vi "Add New Waypoint.vi"(8 "Error In":errorcluster, 9 "Altitude (m)":sgl, 10 "Lon":sgl, 11 "Lat":sgl) -> (0 "Error Out":errorcluster)   [LabVIEW 2014]
uses:
  Aircraft Information/Sub VI/Selected Aircraft/SubVI/Get Selected Aircraft.vi
  Aircraft Information/Sub VI/Get Aircraft Waypoints.vi
  FGV/Methods/Get Waypoint type.vi
  Aircraft Information/Sub VI/Set Aircraft Waypoints.vi
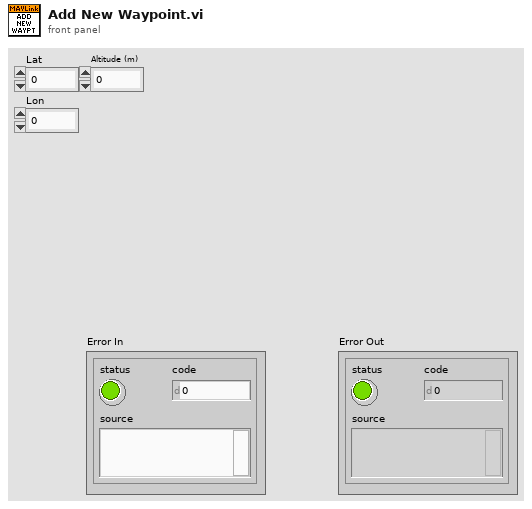
[diagram p1: front panel]
types:
  T1 = typedef "MAVLINK Mav Frame.ctl" = enum8{"GLOBAL", "LOCAL NED", "MISSION", "GLOBAL RELATIVE ALT", "LOCAL ENU", "GLOBAL INT", "GLOBAL RELATIVE ALT INT", "LOCAL OFFSET NED", "BODY NED", "BODY OFFSET NED", "GLOBAL TERRAIN ALT", "GLOBAL TERRAIN ALT INT"}
  T2 = cluster{"target_system":u8, "target_component":u8, "sequence":u16, "frame":T1, "command":u16, "current":bool, "autocontinue":bool, "param1":sgl, "param2":sgl, "param3":sgl, "param4":sgl, "x":sgl, "y":sgl, "z":sgl}[]
  T3 = typedef "Waypoint Type.ctl" = enum16{"PASS-THROUGH", "INSPECT", "CIRCUMNAVIGATE"}
  T4 = typedef "MAVLINK Mission Item.ctl" = cluster{"target_system":u8, "target_component":u8, "sequence":u16, "frame":T1, "command":u16, "current":bool, "autocontinue":bool, "param1":sgl, "param2":sgl, "param3":sgl, "param4":sgl, "Lat":sgl, "Lon":sgl, "Altitude (m)":sgl}
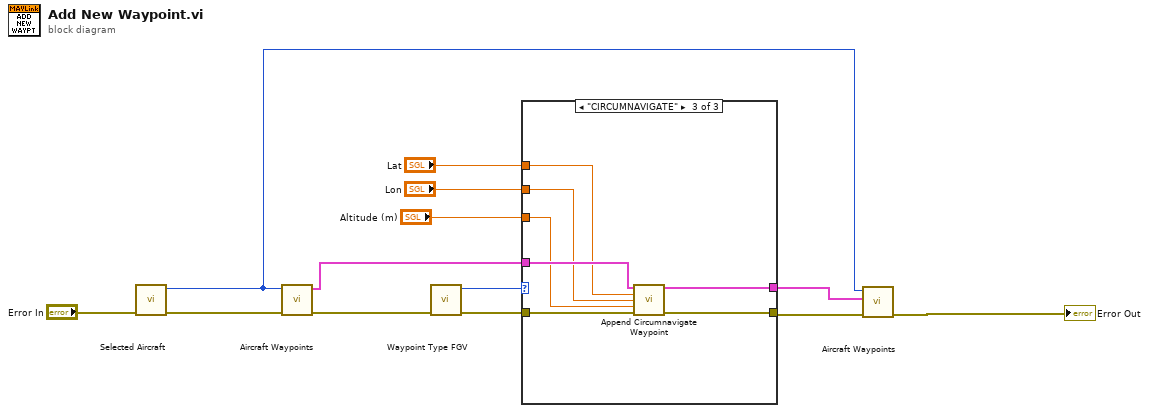
[diagram p0: block diagram]
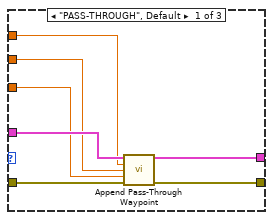
[diagram p2: hidden frame]
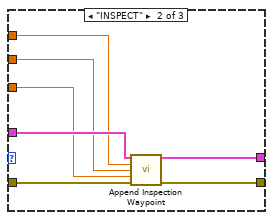
[diagram p3: hidden frame]
diagram:
  n1 = call-poly "Selected Aircraft.vi"("Error In"="Error In") -> ("Error Out"=w12:errorcluster, "Selected Aircraft ID Out"=w2:u8)  [unwired: 9 in]
  n2 = call-poly "Aircraft Waypoints.vi"("Error In"=w12, "Aircraft ID"=w2) -> ("Error Out"=w11:errorcluster, "Waypoints Out"=w9:T2)  [unwired: 8 in]
  n3 = call-poly "Waypoint Type FGV.vi"("Error In"=w11) -> ("Error Out"=w8:errorcluster, "Waypoint Type Out"=w10:T3)  [unwired: 9 in]
  n4 = case shown="\"CIRCUMNAVIGATE\"" w10 {
    tunnel: w9 -> [w20 w24 w31]
    tunnel: w8 -> [w19 w27 w34]
    tunnel: [w18 w26 w33] -> w4
    tunnel: "Lat" -> [w17 w23 w30]
    tunnel: "Lon" -> [w16 w22 w29]
    tunnel: "Altitude (m)" -> [w15 w21 w28]
    tunnel: [w14 w25 w32] -> w3
    frame "PASS-THROUGH", Default {
      n5 = call "Append Pass-Through Waypoint.vi"("Waypoint Array In"=w20, "Lat"=w17, "Lon"=w16, "Altitude (m)"=w15, "Error In"=w19) -> ("appended array"=w14:T4[], "Error Out"=w18:errorcluster)  [unwired: 9 in]
    }
    frame "INSPECT" {
      n6 = call "Append Inspection Waypoint.vi"("Waypoint Array In"=w24, "Lat"=w23, "Lon"=w22, "Altitude (m)"=w21, "Error In"=w27) -> ("appended array"=w25:T4[], "Error Out"=w26:errorcluster)  [unwired: 9 in]
    }
    frame "CIRCUMNAVIGATE" {
      n7 = call "Append Circumnavigate Waypoint.vi"("Waypoint Array In"=w31, "Lat"=w30, "Lon"=w29, "Altitude (m)"=w28, "Error In"=w34) -> ("appended array"=w32:T4[], "Error Out"=w33:errorcluster)  [unwired: 9 in]
    }
  }
  n8 = call-poly "Aircraft Waypoints.vi"("Error In"=w4, "Waypoints In"=w3, "Aircraft ID"=w2) -> ("Error Out"=→"Error Out":errorcluster)  [unwired: 8 in]
